vi "Close UniCyRO Sim.vi"(8 "error in (no error)":errorcluster, 11 "UniCyRO_Host_Sim in":refnum<class "UniCyRO_Host_Sim.lvclass">) -> (0 "error out":errorcluster)   [LabVIEW 2012, in "UniCyRO.lvlib" / "UniCyRO_Host_Sim.lvclass"]
uses:
  UniCyRO_Host_Sim.lvclass
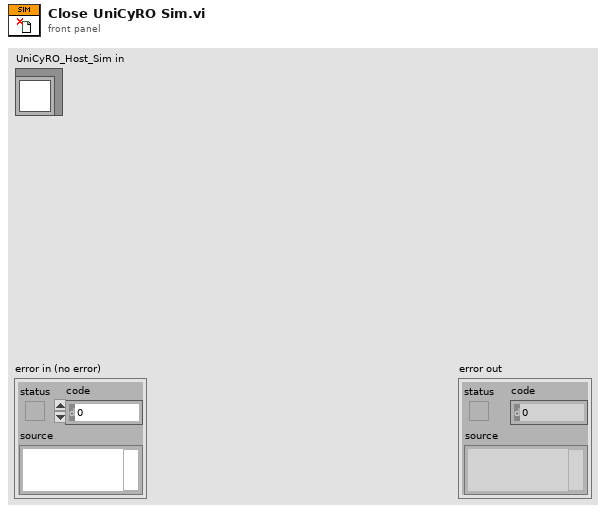
[diagram p1: front panel]
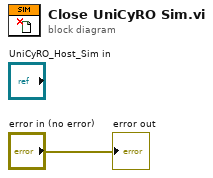
[diagram p0: block diagram]
diagram:
  "error out" <- "error in (no error)"
